vi "3d array testMOD1SlowFill.vi"() -> ()   [LabVIEW 2011]
panel:
  in  "Stop Button":bool
  out "Intensity Slice":sgl[][](array[numeric])
  out "Array 3D":sgl[][][](array[numeric])
  in  "XY Plot Depth":u16(ring) items=["0", "1", "2", "3", "4"]
  in  "Plot":u16(ring) items=["XY", "X cross", "Y cross"]
  out "Intensity Graph":sgl[][](graph)
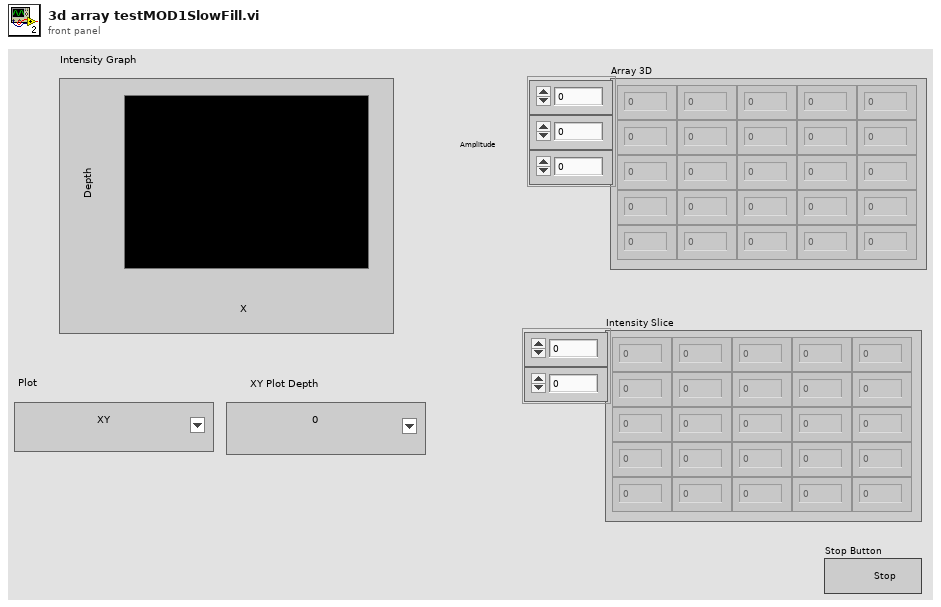
[diagram p1: front panel]
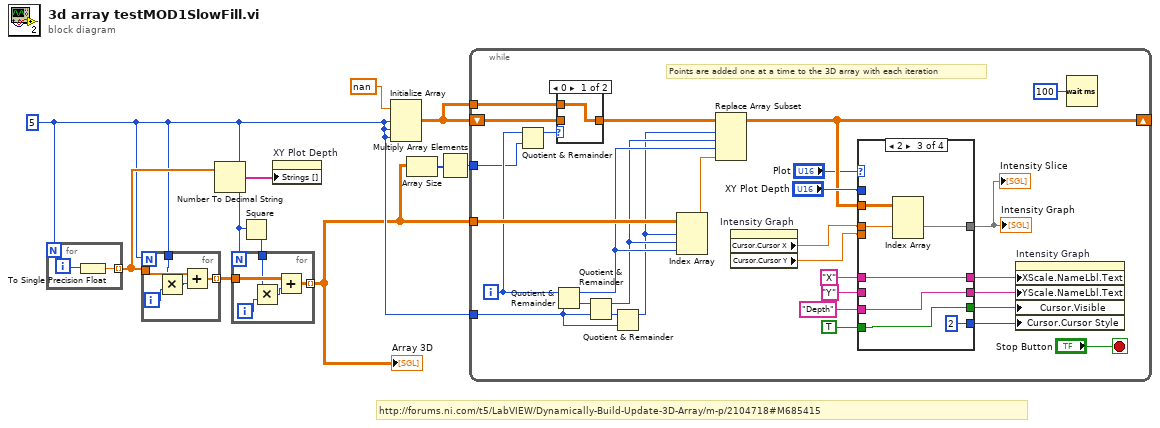
[diagram p0: block diagram]
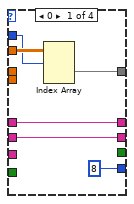
[diagram p2: hidden frame]
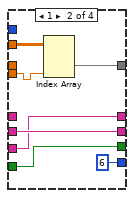
[diagram p3: hidden frame]
diagram:
  w6 = 5
  # "http://forums.ni.com/t5/LabVIEW/Dynamically-Build-Update-3D-Array/m-p/2104718#M685415"
  n1 = for {
    N: w6 -> [_]
    tunnel: [w12] -> w9 mode=indexing
    i -> [w11]
    n2 = To Single Precision Float(number=w11) -> (single precision float=w12:sgl)
  }
  n3 = for {
    N: w6 -> [_]
    tunnel: [w16] -> w8 mode=indexing
    tunnel: w9 -> [w17]
    tunnel: w6 -> [w13]
    i -> [w15]
    n4 = Multiply(x=w13, y=w15) -> (x*y=w14:i32)
    n5 = Add(x=w17, y=w14) -> (x+y=w16:sgl[])
  }
  n6 = Number To Decimal String(number=w9) -> (decimal integer string=w10:string[])  [unwired: 1 in]
  n7 = Square(x=w6) -> (x^2=w4:i32)
  n8 = for {
    N: w6 -> [_]
    tunnel: w8 -> [w22]
    tunnel: [w21] -> w1 mode=indexing
    tunnel: w4 -> [w19]
    i -> [w20]
    n9 = Multiply(x=w19, y=w20) -> (x*y=w18:i32)
    n10 = Add(x=w22, y=w18) -> (x+y=w21:sgl[][])
  }
  "Array 3D" <- w1
  n11 = property on="XY Plot Depth" class="Ring (strict)"("Strings []"=w10) -> ()  [unwired: 2 in, 2 out]
  n12 = Initialize Array(sgl nan ("element"), w6, w6, w6) -> (w5:sgl[][][])
  n13 = Array Size(array=w1) -> (size(s)=w2:i32[])
  n14 = Multiply Array Elements(1:w2) -> (0:w3:i32)
  n15 = while {
    shift-right: [w26] -> _
    shift-left: w5 -> [w46]
    tunnel: w6 -> [w38]
    tunnel: w1 -> [w49]
    tunnel: w5 -> [w45]
    tunnel: w3 -> [w37]
    i -> [w44]
    stop <- "Stop Button" stop-if-true
    # "Points are added one at a time to the 3D array with each iteration"
    n16 = Quotient & Remainder(x=w44, y=w37) -> (x-y*floor(x/y)=w43:i32)  [unwired: 1 out]
    n17 = Quotient & Remainder(x=w44, y=w38) -> (x-y*floor(x/y)=w42:i32, floor(x/y)=w50:i32)
    n18 = case shown="0" w43 {
      tunnel: [w73 w74] -> w47
      tunnel: w46 -> [_ w74]
      tunnel: w45 -> [w73 _]
      frame 0 {
      }
      frame Default {
      }
    }
    n19 = Quotient & Remainder(x=w50, y=w38) -> (x-y*floor(x/y)=w41:i32, floor(x/y)=w40:i32)
    n20 = Quotient & Remainder(x=w40, y=w38) -> (x-y*floor(x/y)=w39:i32)  [unwired: 1 out]
    n21 = Index Array(array=w49, index (dim 0)=w39, index (dim 1)=w41, index (dim 2)=w42) -> (element=w48:sgl)
    n22 = Replace Array Subset(array=w47, new element=w48, index (dim 0)=w39, index (dim 1)=w41, index (dim 2)=w42) -> (w26:sgl[][][])
    n23 = property on="Intensity Graph" class="IntGraph (strict)"() -> ("Cursor.Cursor X"=w27:dbl, "Cursor.Cursor Y"=w23:dbl)  [unwired: 2 in, 2 out]
    n24 = case shown="2" "Plot" {
      tunnel: w26 -> [w58 w65 w72 _]
      tunnel: [w57 w64 w71 _] -> w24
      tunnel: "XY Plot Depth" -> [w54 _ _ _]
      tunnel: [w56 w62 w69 _] -> w36
      tunnel: w23 -> [_ w59 _ _]
      tunnel: [w55 w63 w70 _] -> w35
      tunnel: "X" ("X Scale.Name Label.Text") -> [w56 _ w69 _]
      tunnel: "Y" ("X Scale.Name Label.Text") -> [w55 w63 _ _]
      tunnel: "Depth" ("Y Scale.Name Label.Text") -> [_ w62 w70 _]
      tunnel: [u8 8 ("Cursor.Cursor Style") u8 6 ("Cursor.Cursor Style") u8 2 ("Cursor.Cursor Style") _] -> w31
      tunnel: [_ w60 w67 _] -> w30
      tunnel: TRUE -> [_ w60 w67 _]
      tunnel: w27 -> [_ _ w66 _]
      frame 0 {
        n25 = Index Array(array=w58, index (dim 0)=w54) -> (element=w57:sgl[][])  [unwired: 2 in]
      }
      frame 1 {
        n26 = Index Array(array=w65, index (dim 2)=w59) -> (element=w64:sgl[][])  [unwired: 2 in]
      }
      frame 2 {
        n27 = Index Array(array=w72, index (dim 1)=w66) -> (element=w71:sgl[][])  [unwired: 2 in]
      }
      frame Default {
      }
    }
    "Intensity Graph" <- w24
    "Intensity Slice" <- w24
    n28 = property on="Intensity Graph" class="IntGraph (strict)"("XScale.NameLbl.Text"=w36, "YScale.NameLbl.Text"=w35, "Cursor.Visible"=w30, "Cursor.Cursor Style"=w31) -> ()  [unwired: 2 in, 2 out]
    n29 = Wait (ms)(milliseconds to wait=u32 100) -> ()  [unwired: 1 out]
  }
